vi "GetType.vi"(8 "error in (no error)":errorcluster, 11 "Configure Sparse Marker [SM] Msg in":refnum<class "Configure Sparse Marker [SM] Msg.lvclass">) -> (0 "error out":errorcluster, 2 "Data Sample":variant, 3 "Configure Sparse Marker [SM] Msg out":refnum<class "Configure Sparse Marker [SM] Msg.lvclass">)   [LabVIEW 2014, in "CS++Fgen.lvlib" / "Configure Sparse Marker [SM] Msg.lvclass"]
doc: "This VI delivers a sample of the data type format the message expects."
uses:
  Configure Sparse Marker [SM] Msg.lvclass
  Configure Sparse Marker [SM] Msg.lvclass/Configure Sparse Marker [SM] Msg.ctl
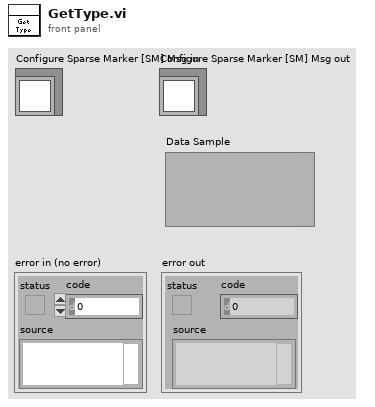
[diagram p1: front panel]
types:
  T1 = cluster{"Marker Name (\"\")":string, "Destination Terminal (None)":string, "Number Indexes":i64, "Waveform Handle":i32, "Indexes Array":i64[]}
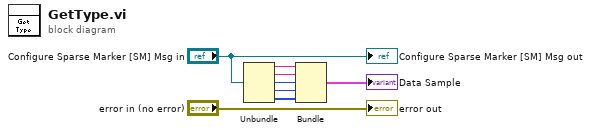
[diagram p0: block diagram]
diagram:
  n1 = Unbundle("Configure Sparse Marker [SM] Msg in") -> (w6:string, w5:string, w2:i64, w3:i32, w4:i64[])
  n2 = Bundle("Marker Name (\"\")"=w6, "Destination Terminal (None)"=w5, "Number Indexes"=w2, "Waveform Handle"=w3, "Indexes Array"=w4) -> (→"Data Sample":T1)  [unwired: 1 in]
  "error out" <- "error in (no error)"
  "Configure Sparse Marker [SM] Msg out" <- "Configure Sparse Marker [SM] Msg in"
